vi "WPI_GyroGetAngle.vi"(8 "error in (no error)":errorcluster, 11 "GyroDevRef":T1) -> (0 "error out":errorcluster, 1 "Angular Rate":dbl, 2 "Angle":dbl, 3 "GyroDevRef":T1)   [LabVIEW 2013]
doc: "Returns the angle, in degrees, from the original heading that the robot is currently facing.\n\nThis software is licensed. Open the labview\\readme\\WPI Robotics Library Open Source License.txt file for more information."
uses:
  <vilib>/Rock Robotics/WPI/Gyro/WPI_GyroDevRef.ctl
  <vilib>/Rock Robotics/SystemInterfaces/Typedef/FPGA_TypedefAnalogModule.ctl
  <vilib>/Rock Robotics/SystemInterfaces/AI/FPGA_AIChannel.ctl
  <vilib>/Rock Robotics/SystemInterfaces/AI/FPGA_AIGyroChannel.ctl
  <instrlib>/Sparkfun Atomic IMU/HAIOL/Sparkfun Atomic IMU.lvclass
  <instrlib>/Honeywell Compass HMC6343/HAIOL/Honeywell Compass HMC6343.lvclass
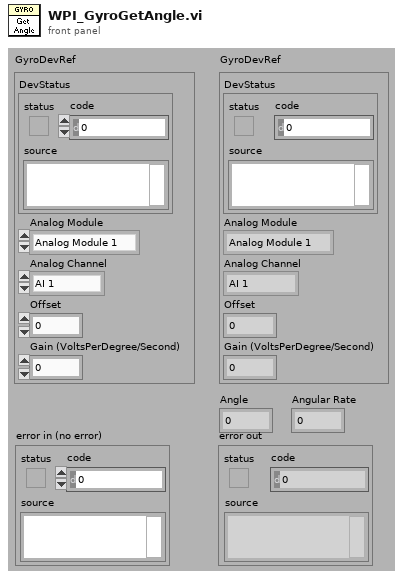
[diagram p1: front panel]
types:
  T1 = typedef "WPI_GyroDevRef.ctl" = cluster{"DevStatus":errorcluster, "Analog Module":T2, "Analog Channel":T3, "Offset":dbl, "Gain (VoltsPerDegree/Second)":dbl}
  T2 = typedef "FPGA_TypedefAnalogModule.ctl" = enum16{"Analog Module 1", "Analog Module 2"}
  T3 = typedef "FPGA_AIChannel.ctl" = enum8{"AI 1", "AI 2", "AI 3", "AI 4", "AI 5", "AI 6", "AI 7", "AI 8", "Invalid"}
  T4 = typedef "FPGA_AIGyroChannel.ctl" = enum8{"AI 1", "AI 2", "Invalid"}
  T5 = cluster{"Pitch (deg/s)":dbl, "Roll (deg/s)":dbl, "Yaw (deg/s)":dbl}
  T6 = cluster{"Head (deg)":dbl, "Pitch (deg)":dbl, "Roll (deg)":dbl}
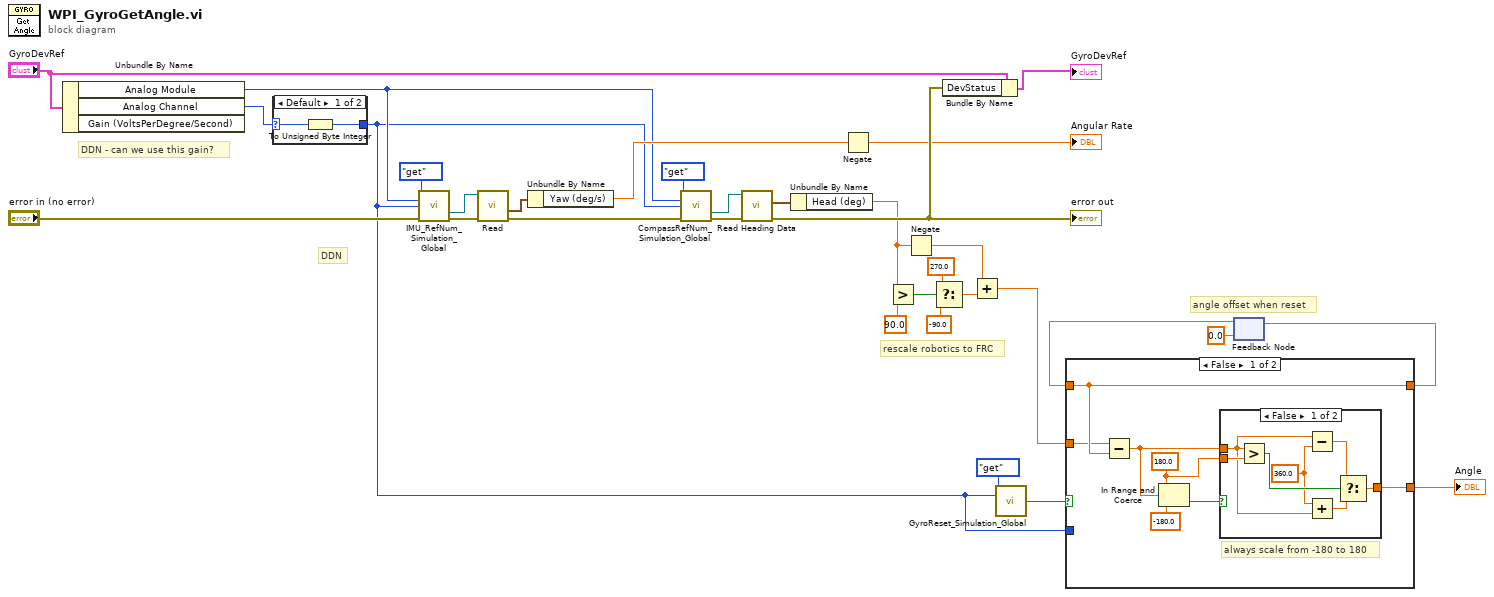
[diagram p0: block diagram]
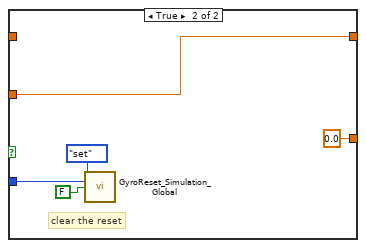
[diagram p3: hidden frame]
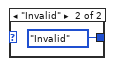
[diagram p4: hidden frame]
diagram:
  # "angle offset when reset"
  # "rescale robotics to FRC"
  # "DDN"
  # "DDN - can we use this gain?"
  n1 = Unbundle By Name("GyroDevRef") -> ("Analog Module"=w21:T2, "Analog Channel"=w29:T3)  [unwired: 1 out]
  n2 = case shown="Default" w29 {
    selector: w29 -> [w34 _]
    tunnel: [w33 FPGA_AIGyroChannel."Invalid" ("Analog Channel")] -> w1
    frame Default {
      n3 = To Unsigned Byte Integer(number=w34) -> (unsigned 8bit integer=w33:u8)
    }
    frame "Invalid" {
    }
  }
  n4 = call <vilib>:"IMU_RefNum_Simulation_Global.vi"("menu"=enum16{"set", "get", "delete"}."get", "Analog Module (Module 1)"=w21, "Analog Channel"=w1, "error in (no error)"="error in (no error)") -> ("Sparkfun Atomic IMU Get"=w26:refnum<class "Sparkfun Atomic IMU.lvclass">, "error out"=w27:errorcluster)  [unwired: 10 in]
  n5 = call-dynamic "Read.vi"("error in (no error)"=w27, "Sparkfun Atomic IMU in"=w26) -> ("error out"=w23:errorcluster, "Gyros Data"=w25:T5)  [unwired: 6 in, 2 out]
  n6 = Unbundle By Name(w25) -> ("Yaw (deg/s)"=w24:dbl)
  n7 = call <vilib>:"CompassRefNum_Simulation_Global.vi"("menu"=enum16{"set", "get", "delete"}."get", "Analog Module (Module 1)"=w21, "Analog Channel"=w1, "error in (no error)"=w23) -> ("Honeywell Compass HMC6343 Get"=w17:refnum<class "Honeywell Compass HMC6343.lvclass">, "error out"=w19:errorcluster)  [unwired: 10 in]
  n8 = call-dynamic "Read Heading Data.vi"("error in (no error)"=w19, "Honeywell Compass HMC6343"=w17) -> ("error out"=w22:errorcluster, "Heading Data"=w18:T6)  [unwired: 7 in, 1 out]
  "error out" <- w22
  n9 = Unbundle By Name(w18) -> ("Head (deg)"=w9:dbl)
  n10 = Negate(x=w24) -> (-x=→"Angular Rate":dbl)
  n11 = Greater?(x=w9, y=90.0) -> (0:w14:bool)
  n12 = Negate(x=w9) -> (-x=w12:dbl)
  n13 = Select(t=270.0, s=w14, f=-90.0) -> (s? t:f=w13:dbl)
  n14 = Bundle By Name(cluster="GyroDevRef", "DevStatus"=w22) -> (→"GyroDevRef":T1)
  n15 = Add(x=w12, y=w13) -> (x+y=w3:dbl)
  n16 = call <vilib>:"GyroReset_Simulation_Global.vi"("menu"=enum16{"set", "get", "delete"}."get", "Gyro Channel"=w1) -> ("reset out"=w7:bool)  [unwired: 12 in, 1 out]
  n17 = feedback #1(0.0 ("In Gauge")) -> (w5:dbl)
  n18 = case shown="False" w7 {
    tunnel: w5 -> [w38 _]
    tunnel: [w38 w55] -> w4
    tunnel: w3 -> [w37 w55]
    tunnel: [w36 0.0] -> w2
    tunnel: w1 -> [_ w52]
    frame False {
      w42 = 180.0 ("y")
      # "always scale from -180 to 180"
      n19 = Subtract(x=w37, y=w38) -> (x-y=w39:dbl)
      n20 = In Range and Coerce(upper limit=w42, x=w39, lower limit=-180.0 ("y")) -> (In Range?=w41:bool)  [unwired: 1 out]
      n21 = case shown="False" w41 {
        tunnel: [w48 w50] -> w36
        tunnel: w39 -> [w44 w50]
        tunnel: w42 -> [w49 _]
        frame False {
          w43 = 360.0 ("y")
          n22 = Greater?(x=w44, y=w49) -> (0:w47:bool)
          n23 = Subtract(x=w44, y=w43) -> (x-y=w46:dbl)
          n24 = Add(x=w43, y=w44) -> (x+y=w45:dbl)
          n25 = Select(t=w46, s=w47, f=w45) -> (s? t:f=w48:dbl)
        }
        frame True {
        }
      }
    }
    frame True {
      # "clear the reset"
      n26 = call <vilib>:"GyroReset_Simulation_Global.vi"("menu"=enum16{"set", "get", "delete"}."set", "Gyro Channel"=w52, "reset in"=FALSE) -> ()  [unwired: 11 in, 2 out]
    }
  }
  "Angle" <- w2
  n27 = feedback-in #1(w4) -> ()
